vi "Read waveform data sub.vi"(6 "错误输入（无错误）":errorcluster, 8 "读取数据大小":u32, 9 "VISA资源名称":refnum<visa-resource-name>) -> (0 "错误输出":errorcluster, 1 "波形数据":u8[](array[numeric]), 2 "返回数":u32, 3 "VISA资源名称输出":refnum<visa-resource-name>)   [LabVIEW 2015, in "ZhiYuan ZDS Series for TCP.lvlib"]
uses:
  ZhiYuan ZDS Series for TCP.lvlib
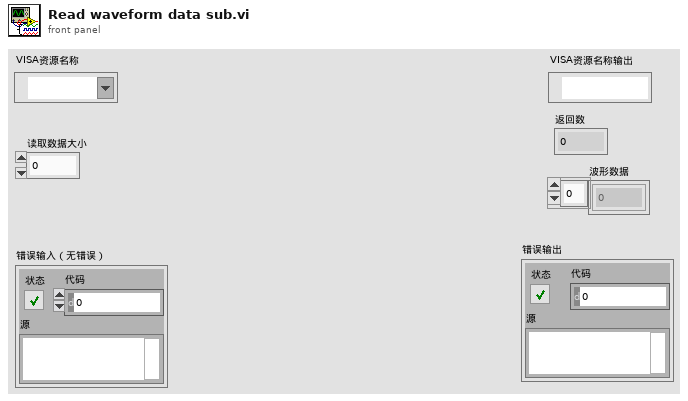
[diagram p1: front panel]
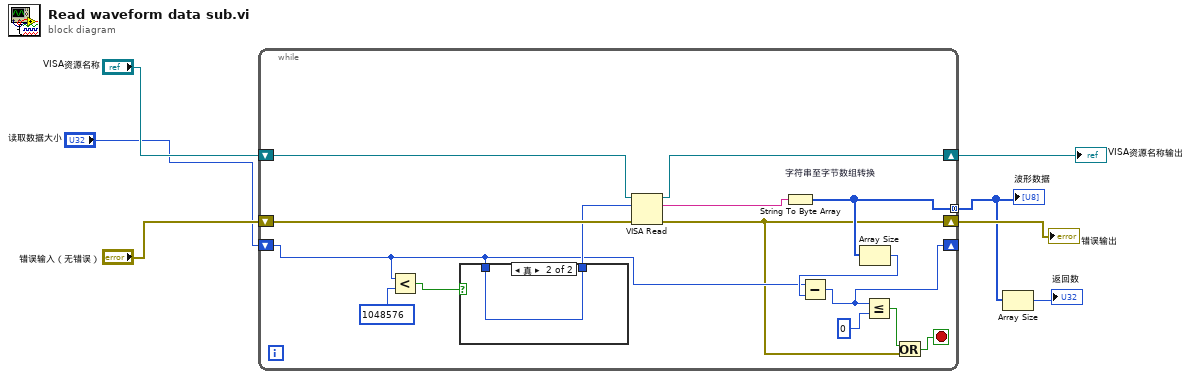
[diagram p0: block diagram]
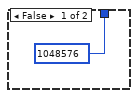
[diagram p2: hidden frame]
diagram:
  n1 = while {
    shift-right: [w21] -> w6
    shift-left: "VISA资源名称" -> [w22]
    shift-right: [w10] -> w4
    shift-left: "错误输入（无错误）" -> [w20]
    tunnel: [w14] -> w3 mode=concatenating
    shift-right: [w11] -> _
    shift-left: "读取数据大小" -> [w12]
    stop <- w8 stop-if-true
    n2 = Less?(x=w12, y=1048576) -> (x < y?=w16:bool)
    n3 = case shown="真" w16 {
      tunnel: [1048576 w24] -> w19
      tunnel: w12 -> [_ w24]
      frame False {
      }
      frame True {
      }
    }
    n4 = VISA Read(VISA resource name=w22, byte count=w19, error in (no error)=w20) -> (VISA resource name out=w21:refnum<visa-resource-name>, read buffer=w18:string, error out=w10:errorcluster)  [unwired: 1 out]
    n5 = String To Byte Array "字符串至字节数组转换"(string=w18) -> (unsigned byte array=w14:u8[])
    n6 = Array Size(array=w14) -> (size(s)=w13:i32)
    n7 = Subtract(x=w12, y=w13) -> (x-y=w11:u32)
    n8 = Less Or Equal?(x=w11, y=0) -> (x <= y?=w9:bool)
    n9 = Or(x=w9, y=w10) -> (x .or. y?=w8:bool)
  }
  "VISA资源名称输出" <- w6
  "错误输出" <- w4
  "波形数据" <- w3
  n10 = Array Size(array=w3) -> (size(s)=→"返回数":i32)
